vi "chart axis set interval tick.vi"(8 "error in (no error)":errorcluster, 10 "unit":u16, 11 "axis":u32) -> (0 "error out":errorcluster)   [LabVIEW 8.6]
doc: "void chart_axis_set_interval_tick(lxw_chart_axis axis, uint16_t unit);"
uses:
  pending_lvxlsxwriter/xlsxwriter.dll
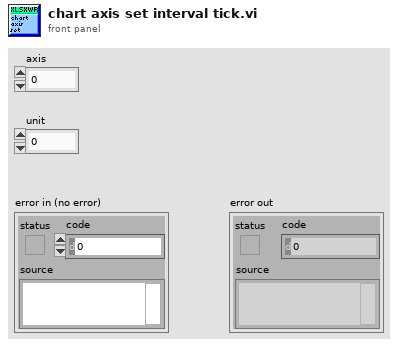
[diagram p1: front panel]
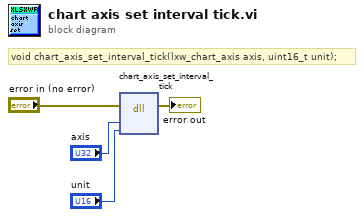
[diagram p0: block diagram]
diagram:
  # "void chart_axis_set_interval_tick(lxw_chart_axis axis, uint16_t unit);"
  n1 = dll-call lib="C:/Users/WDAGUtilityAccount/Desktop/pending_lvxlsxwriter/xlsxwriter.*" fn="chart_axis_set_interval_tick"(error in="error in (no error)", "axis"="axis", "unit"="unit") -> (error out=→"error out":errorcluster)  [unwired: 5 in, 1 out]
